vi "init data structures.vi"(8 "error in":errorcluster, 9 "data allocations":T1, 10 "shared memory configuration":refnum<class "shared memory configuration.lvclass">, 11 "shared memory runtime in":refnum<class "shared memory runtime.lvclass">) -> (0 "error out":errorcluster, 3 "shared memory runtime out":refnum<class "shared memory runtime.lvclass">)   [LabVIEW 2013, in "shared memory runtime.lvclass"]
uses:
  shared memory runtime.lvclass
  configuration/shared memory configuration.lvclass
  <vilib>/NI/Tag Bus Module Framework/channel/data tables.ctl
  <vilib>/NI/Tag Bus/dictionary/data dictionary.lvclass
  <vilib>/NI/Tag Bus/dictionary table pair.ctl
  <vilib>/NI/Tag Bus/table/data table.ctl
  configuration/shared memory configuration.lvclass/shared memory configuration.ctl
  <vilib>/NI/Tag Bus/tag/tag descriptor.lvclass/tag descriptor.ctl
  <vilib>/NI/Tag Bus Module Framework/channel/TBM channel.lvclass/TBM channel.ctl
  shared memory runtime.lvclass/shared memory runtime.ctl
  shared memory module runtime.ctl
  <vilib>/NI/Tag Bus Module Framework/channel/channel classification.ctl
  <vilib>/NI/Tag Bus/tag/Data Type.ctl
  <vilib>/National Instruments/Shared Memory Library for Linux RT/Controls/Shared Memory Class Reference.ctl
  <vilib>/National Instruments/Shared Memory Library for Linux RT/Classes/Shared Memory/Shared Memory.lvclass
  <vilib>/National Instruments/Shared Memory Library for Linux RT/Controls/File Mode.ctl
  configuration/Read Write Directory.vi
  configuration/Read Read Directory.vi
  configuration/Read lines.vi
  <vilib>/NI/Tag Bus/tag/read tag name.vi
  <vilib>/NI/Tag Bus/dictionary/locate tag.vi
  <vilib>/NI/Tag Bus Module Framework/channel/TBM channel.lvclass
  <vilib>/NI/Tag Bus/tag/tag descriptor.lvclass
  <vilib>/National Instruments/Shared Memory Library for Linux RT/Shared Memory.lvlib
  <vilib>/NI/Tag Bus/table/data table.lvlib
  <vilib>/NI/Tag Bus/tag bus.lvlib
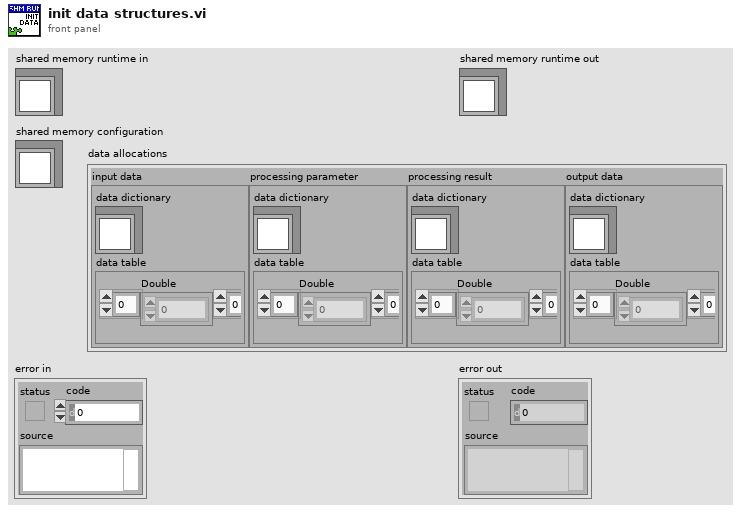
[diagram p1: front panel]
types:
  T1 = typedef "TBM channel.lvclass/data tables.ctl" = cluster{"input data":T2, "processing parameter":T2, "processing result":T2, "output data":T2}
  T2 = typedef "tag bus.lvlib/dictionary table pair.ctl" = cluster{"data dictionary":refnum<class "data dictionary.lvclass">, "data table":T3}
  T3 = typedef "tag bus.lvlib/data table.lvlib/data table.ctl" = cluster{"Double":dbl[], "Single":sgl[], "I64":i64[], "I32":i32[], "I16":i16[], "I8":i8[], "U64":u64[], "U32":u32[], "U16":u16[], "U8":u8[], "Boolean":bool[], "String":string[], "Array of Double":cluster{"DBL Array":dbl[]}[], "Array of Single":cluster{"SGL Array":sgl[]}[], "Array of I64":cluster{"I64 Array":i64[]}[], "Array of I32":cluster{"I32 Array":i32[]}[], "Array of I16":cluster{"I16 Array":i16[]}[], "Array of I8":cluster{"I8 Array":i8[]}[], "Array of U64":cluster{"U64 Array":u64[]}[], "Array of U32":cluster{"U32 Array":u32[]}[], "Array of U16":cluster{"U16 Array":u16[]}[], "Array of U8":cluster{"U8 Array":u8[]}[], "Array of Boolean":cluster{"Boolean Array":bool[]}[], "Array of String":cluster{"String Array":string[]}[]}
  T4 = typedef "shared memory configuration.lvclass/Line.ctl" = cluster{"name":string, "data type":T5, "channel":refnum<class "TBM channel.lvclass">}
  T5 = typedef "tag bus.lvlib/tag descriptor.lvclass/Data Type.ctl" = enum16{"Double", "Single", "I64", "I32", "I16", "I8", "U64", "U32", "U16", "U8", "Boolean", "String", "Array of Double", "Array of Single", "Array of I64", "Array of I32", "Array of I16", "Array of I8", "Array of U64", "Array of U32", "Array of U16", "Array of U8", "Array of Boolean", "Array of String"}
  T6 = typedef "Shared Memory.lvlib/File Mode.ctl" = enum16{"open", "create/replace"}
  T7 = typedef "shared memory runtime.lvclass/shared memory module runtime.ctl" = cluster{"channel classification":T8, "data type":T5, "pointer to shared memory":u64, "number of elements":u64, "data dictionary index":cluster{i32[]}, "shared memory":T9}
  T8 = typedef "TBM channel.lvclass/channel classification.ctl" = enum16{"input data", "output data", "processing parameter", "processing result"}
  T9 = typedef "Shared Memory Class Reference.ctl" = refnum<data-value>
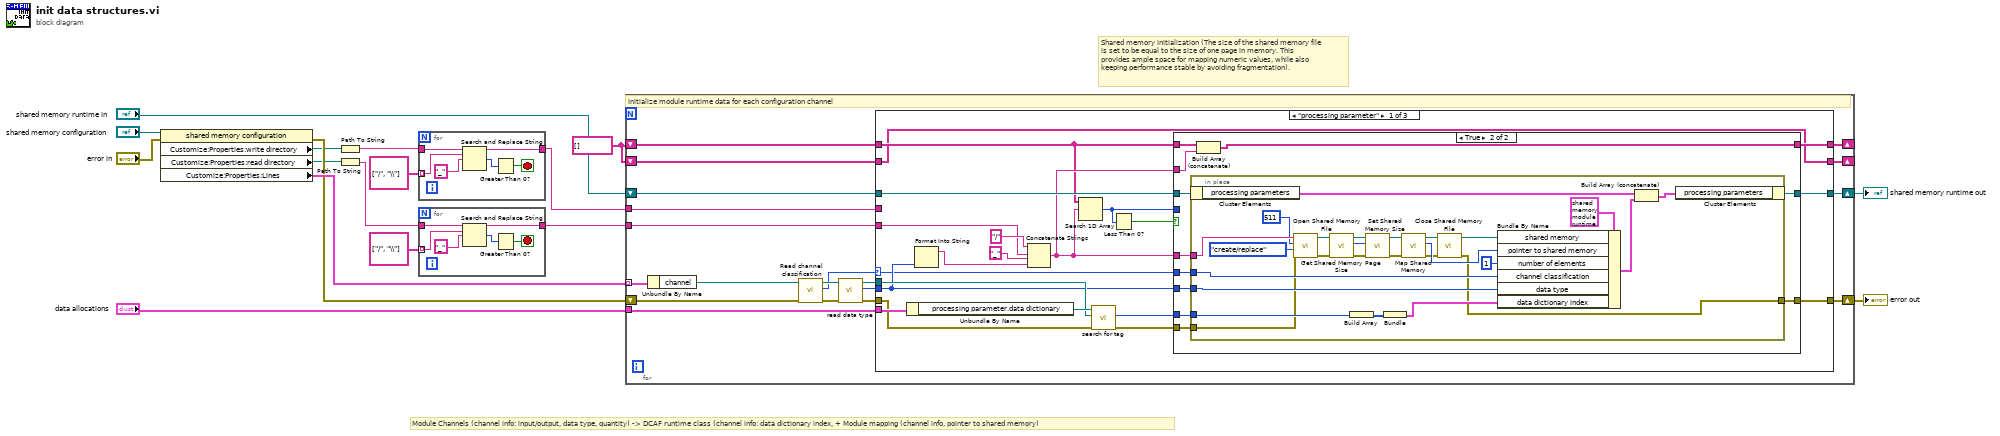
[diagram p0: block diagram]
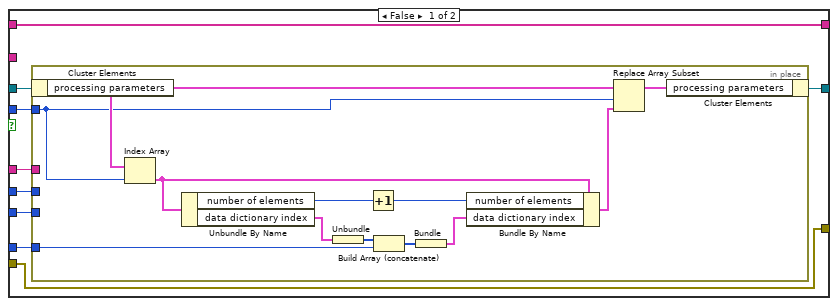
[diagram p2: hidden frame]
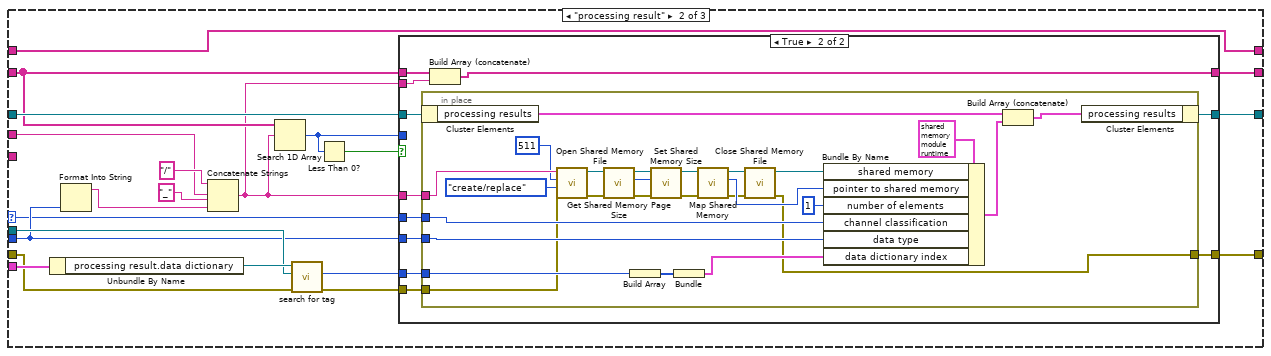
[diagram p3: hidden frame]
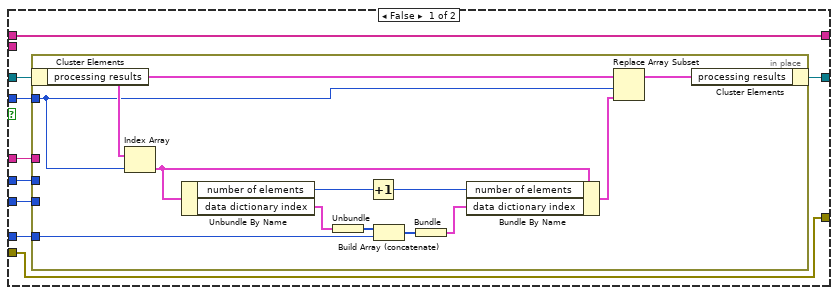
[diagram p4: hidden frame]
diagram:
  w7 = string[] []
  # "Shared memory initialization (The size of the shared memory file is set to be equal to the size of one page in memory. This provides ample space for mapping numeric values, while also keeping performance stable by avoiding fragmentation)."
  # "Module Channels (channel info: input/output, data type, quantity) -> DCAF runtime class (channel info: data dictionary index, + Module mapping (channel info, pointer to shared memory)"
  n1 = property class="shared memory configuration"(reference="shared memory configuration", error in="error in") -> (error out=w3:errorcluster, "Customize:Properties:write directory"=w1:path, "Customize:Properties:read directory"=w2:path, "Customize:Properties:Lines"=w4:T4[])  [unwired: 1 out]
  n2 = Path To String(path=w1) -> (string=w9:string)
  n3 = Path To String(path=w2) -> (string=w11:string)
  n4 = for {
    tunnel: string[] ["/", "\\"] -> [w22] mode=indexing
    tunnel: w9 -> [w23]
    tunnel: [w18] -> w5
    stop <- w19 stop-if-true
    n5 = Search and Replace String(input string=w23, search string=w22, replace string="_" ("replace string (\"\")")) -> (result string=w18:string, number of replacements=w20:i32)  [unwired: 5 in, 2 out]
    n6 = Greater Than 0?(x=w20) -> (x > 0?=w19:bool)
  }
  n7 = for {
    tunnel: string[] ["/", "\\"] -> [w28] mode=indexing
    tunnel: w11 -> [w29]
    tunnel: [w24] -> w6
    stop <- w25 stop-if-true
    n8 = Search and Replace String(input string=w29, search string=w28, replace string="_" ("replace string (\"\")")) -> (result string=w24:string, number of replacements=w26:i32)  [unwired: 5 in, 2 out]
    n9 = Greater Than 0?(x=w26) -> (x > 0?=w25:bool)
  }
  n10 = for {
    tunnel: w4 -> [w47] mode=indexing
    tunnel: "data allocations" -> [w42]
    shift-right: [w37] -> w13
    shift-left: "shared memory runtime in" -> [w38]
    tunnel: w5 -> [w36]
    tunnel: w6 -> [w35]
    shift-right: [w34] -> _
    shift-left: w7 -> [w33]
    shift-right: [w32] -> _
    shift-left: w7 -> [w31]
    shift-right: [w30] -> w12
    shift-left: w3 -> [w39]
    # "Initialize module runtime data for each configuration channel"
    n11 = Unbundle By Name(w47) -> ("channel"=w48:refnum<class "TBM channel.lvclass">)
    n12 = call <vilib>:"Read channel classification.vi"("error in"=w39, "channel in"=w48) -> ("error out"=w45:errorcluster, "channel classification"=w43:T8, "channel out"=w46:refnum<class "TBM channel.lvclass">)  [unwired: 7 in]
    n13 = call <vilib>:"read data type.vi"("error in"=w45, "system tag in"=w46) -> ("error out"=w40:errorcluster, "data type"=w44:T5, "system tag out"=w41:refnum<class "TBM channel.lvclass">)  [unwired: 7 in]
    n14 = case shown="\"processing parameter\"" w43 {
      selector: w43 -> [w59 w138 _]
      tunnel: w44 -> [w60 w139 _]
      tunnel: w42 -> [w69 w148 _]
      tunnel: w41 -> [w67 w146 _]
      tunnel: w40 -> [w66 w145 w207]
      tunnel: w38 -> [w65 w144 w210]
      tunnel: [w64 w143 w210] -> w37
      tunnel: w36 -> [_ w128 _]
      tunnel: w35 -> [w49 _ _]
      tunnel: [w52 w134 w208] -> w34
      tunnel: w33 -> [w52 w136 w208]
      tunnel: [w53 w137 w209] -> w32
      tunnel: w31 -> [w54 w137 w209]
      tunnel: [w50 w129 w207] -> w30
      frame "processing parameter" {
        n15 = Unbundle By Name(w69) -> ("processing parameter.data dictionary"=w68:refnum<class "data dictionary.lvclass">)
        n16 = Format Into String(w60) -> (resulting string=w61:string)  [unwired: 3 in, 1 out]
        n17 = Concatenate Strings("/" ("string"), w49, "_" ("shared memory name"), w61) -> (w58:string)
        n18 = Search 1D Array(1D array=w54, element=w58) -> (index of element=w56:i32)  [unwired: 1 in]
        n19 = call <vilib>:"search for tag.vi"("error in"=w66, "system tag"=w67, "data dictionary in"=w68) -> ("error out"=w51:errorcluster, "index"=w55:i32)  [unwired: 6 in, 1 out]
        n20 = Less Than 0?(x=w56) -> (x < 0?=w57:bool)
        n21 = case shown="True" w57 {
          tunnel: w55 -> [w78 w101]
          tunnel: w65 -> [w77 w100]
          tunnel: [w76 w99] -> w64
          tunnel: w60 -> [w75 w98]
          tunnel: w59 -> [w74 w97]
          tunnel: w58 -> [w73 w96]
          tunnel: w58 -> [_ w95]
          tunnel: [w71 w94] -> w53
          tunnel: w56 -> [w72 _]
          tunnel: w54 -> [w71 w93]
          tunnel: w51 -> [w70 w92]
          tunnel: [w70 w91] -> w50
          frame False {
            n22 = in-place {
              in-place-border: w78 -> [w81]
              in-place-border: w75 -> [_]
              in-place-border: w73 -> [_]
              in-place-border: w74 -> [_]
              in-place-border: w72 -> [w87]
              n23 = in-place-cluster #1(w77) -> ("processing parameters"=w90:T7[])
              n24 = Index Array(array=w90, index=w87) -> (element=w86:T7)
              n25 = Unbundle By Name(w86) -> ("number of elements"=w85:u64, "data dictionary index"=w83:cluster{i32[]})
              n26 = Unbundle(w83) -> (w82:i32[])
              n27 = Increment(x=w85) -> (x+1=w84:u64)
              n28 = Build Array (concatenate)(w82, w81) -> (w80:i32[])
              n29 = Bundle(w80) -> (w79:cluster{i32[]})  [unwired: 1 in]
              n30 = Bundle By Name(cluster=w86, "number of elements"=w84, "data dictionary index"=w79) -> (w88:T7)
              n31 = Replace Array Subset(array=w90, new element=w88, index=w87) -> (w89:T7[])
              n32 = in-place-cluster #1("processing parameters"=w89) -> (w76:refnum<class "shared memory runtime.lvclass">)
            }
          }
          frame True {
            n33 = in-place {
              in-place-border: w101 -> [w109]
              in-place-border: w98 -> [w126]
              in-place-border: w96 -> [w113]
              in-place-border: w97 -> [w122]
              in-place-border: w92 -> [w107]
              in-place-border: [w104] -> w91
              n34 = in-place-cluster #2(w100) -> ("processing parameters"=w125:T7[])
              n35 = call <vilib>:"Open Shared Memory File.vi"("error in (no error)"=w107, "file mode (default: open)"=File_Mode."create/replace", "permissions (default: 0664)"=u32 511, "shared memory name"=w113) -> ("error out"=w117:errorcluster, "shared memory out"=w121:T9)  [unwired: 6 in]
              n36 = call <vilib>:"Get Shared Memory Page Size.vi"("error in (no error)"=w117, "shared memory in"=w121) -> ("error out"=w116:errorcluster, "page size (bytes)"=w118:u32, "shared memory out"=w120:T9)  [unwired: 7 in]
              n37 = Build Array(w109) -> (w110:i32[])
              n38 = call <vilib>:"Set Shared Memory Size.vi"("error in (no error)"=w116, "size (bytes)"=w118, "shared memory in"=w120) -> ("error out"=w115:errorcluster, "shared memory out"=w119:T9)  [unwired: 7 in]
              n39 = Bundle(w110) -> (w108:cluster{i32[]})  [unwired: 1 in]
              n40 = call <vilib>:"Map Shared Memory.vi"("error in (no error)"=w115, "shared memory in"=w119) -> ("error out"=w105:errorcluster, "pointer to shared memory"=w112:u64, "shared memory out"=w106:T9)  [unwired: 7 in]
              n41 = call <vilib>:"Close Shared Memory File.vi"("error in (no error)"=w105, "shared memory in"=w106) -> ("error out"=w104:errorcluster, "shared memory out"=w102:T9)  [unwired: 8 in]
              n42 = Bundle By Name(cluster=T7 {"channel classification"=enum."input data", "data type"=enum."Double", "pointer to shared memory"=0, "number of elements"=0, "data dictionary index"={[]}, "shared memory"=refnum} ("runtime"), "shared memory"=w102, "pointer to shared memory"=w112, "number of elements"=u64 1 ("quantity"), "channel classification"=w122, "data type"=w126, "data dictionary index"=w108) -> (w124:T7)
              n43 = Build Array (concatenate)(w125, w124) -> (w123:T7[])
              n44 = in-place-cluster #2("processing parameters"=w123) -> (w99:refnum<class "shared memory runtime.lvclass">)
            }
            n45 = Build Array (concatenate)(w93, w95) -> (w94:string[])
          }
        }
      }
      frame "processing result" {
        n46 = Unbundle By Name(w148) -> ("processing result.data dictionary"=w147:refnum<class "data dictionary.lvclass">)
        n47 = Format Into String(w139) -> (resulting string=w140:string)  [unwired: 3 in, 1 out]
        n48 = Concatenate Strings("/" ("string"), w128, "_" ("shared memory name"), w140) -> (w135:string)
        n49 = Search 1D Array(1D array=w136, element=w135) -> (index of element=w132:i32)  [unwired: 1 in]
        n50 = call <vilib>:"search for tag.vi"("error in"=w145, "system tag"=w146, "data dictionary in"=w147) -> ("error out"=w130:errorcluster, "index"=w131:i32)  [unwired: 6 in, 1 out]
        n51 = Less Than 0?(x=w132) -> (x < 0?=w133:bool)
        n52 = case shown="True" w133 {
          tunnel: w131 -> [w157 w180]
          tunnel: w144 -> [w156 w179]
          tunnel: [w155 w178] -> w143
          tunnel: w139 -> [w154 w177]
          tunnel: w138 -> [w153 w176]
          tunnel: w135 -> [w152 w175]
          tunnel: w136 -> [w150 w174]
          tunnel: w135 -> [_ w173]
          tunnel: [w150 w172] -> w134
          tunnel: w132 -> [w151 _]
          tunnel: w130 -> [w149 w171]
          tunnel: [w149 w170] -> w129
          frame False {
            n53 = in-place {
              in-place-border: w157 -> [w160]
              in-place-border: w154 -> [_]
              in-place-border: w152 -> [_]
              in-place-border: w153 -> [_]
              in-place-border: w151 -> [w166]
              n54 = in-place-cluster #3(w156) -> ("processing results"=w169:T7[])
              n55 = Index Array(array=w169, index=w166) -> (element=w165:T7)
              n56 = Unbundle By Name(w165) -> ("number of elements"=w164:u64, "data dictionary index"=w162:cluster{i32[]})
              n57 = Unbundle(w162) -> (w161:i32[])
              n58 = Increment(x=w164) -> (x+1=w163:u64)
              n59 = Build Array (concatenate)(w161, w160) -> (w159:i32[])
              n60 = Bundle(w159) -> (w158:cluster{i32[]})  [unwired: 1 in]
              n61 = Bundle By Name(cluster=w165, "number of elements"=w163, "data dictionary index"=w158) -> (w167:T7)
              n62 = Replace Array Subset(array=w169, new element=w167, index=w166) -> (w168:T7[])
              n63 = in-place-cluster #3("processing results"=w168) -> (w155:refnum<class "shared memory runtime.lvclass">)
            }
          }
          frame True {
            n64 = in-place {
              in-place-border: w180 -> [w188]
              in-place-border: w177 -> [w205]
              in-place-border: w175 -> [w192]
              in-place-border: w176 -> [w201]
              in-place-border: w171 -> [w186]
              in-place-border: [w184] -> w170
              n65 = in-place-cluster #4(w179) -> ("processing results"=w204:T7[])
              n66 = call <vilib>:"Open Shared Memory File.vi"("error in (no error)"=w186, "file mode (default: open)"=File_Mode."create/replace", "permissions (default: 0664)"=u32 511, "shared memory name"=w192) -> ("error out"=w196:errorcluster, "shared memory out"=w200:T9)  [unwired: 6 in]
              n67 = call <vilib>:"Get Shared Memory Page Size.vi"("error in (no error)"=w196, "shared memory in"=w200) -> ("error out"=w195:errorcluster, "page size (bytes)"=w197:u32, "shared memory out"=w199:T9)  [unwired: 7 in]
              n68 = Build Array(w188) -> (w189:i32[])
              n69 = call <vilib>:"Set Shared Memory Size.vi"("error in (no error)"=w195, "size (bytes)"=w197, "shared memory in"=w199) -> ("error out"=w194:errorcluster, "shared memory out"=w198:T9)  [unwired: 7 in]
              n70 = Bundle(w189) -> (w187:cluster{i32[]})  [unwired: 1 in]
              n71 = call <vilib>:"Map Shared Memory.vi"("error in (no error)"=w194, "shared memory in"=w198) -> ("error out"=w185:errorcluster, "pointer to shared memory"=w191:u64, "shared memory out"=w183:T9)  [unwired: 7 in]
              n72 = call <vilib>:"Close Shared Memory File.vi"("error in (no error)"=w185, "shared memory in"=w183) -> ("error out"=w184:errorcluster, "shared memory out"=w182:T9)  [unwired: 8 in]
              n73 = Bundle By Name(cluster=T7 {"channel classification"=enum."input data", "data type"=enum."Double", "pointer to shared memory"=0, "number of elements"=0, "data dictionary index"={[]}, "shared memory"=refnum} ("tag config"), "shared memory"=w182, "pointer to shared memory"=w191, "number of elements"=u64 1 ("quantity"), "channel classification"=w201, "data type"=w205, "data dictionary index"=w187) -> (w203:T7)
              n74 = Build Array (concatenate)(w204, w203) -> (w202:T7[])
              n75 = in-place-cluster #4("processing results"=w202) -> (w178:refnum<class "shared memory runtime.lvclass">)
            }
            n76 = Build Array (concatenate)(w174, w173) -> (w172:string[])
          }
        }
      }
      frame Default {
      }
    }
  }
  "error out" <- w12
  "shared memory runtime out" <- w13
